vi "Get Channel Tag Path.vi"(11 "Waveform":waveform(dbl)) -> (3 "channel path":string)   [LabVIEW 2017, in "Logger.lvclass"]
uses:
  logger/Logger.lvclass
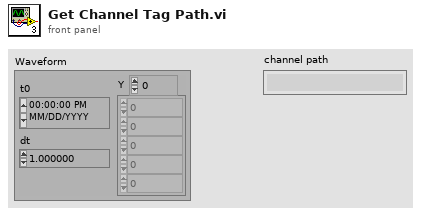
[diagram p1: front panel]
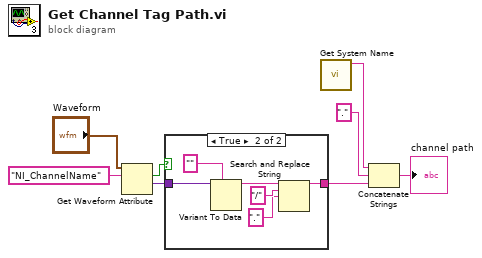
[diagram p0: block diagram]
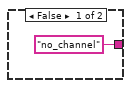
[diagram p2: hidden frame]
diagram:
  n1 = Get Waveform Attribute(6:"NI_ChannelName" ("name"), 7:"Waveform") -> (1:w7:variant, 2:w6:bool)  [unwired: 2 in, 2 out]
  n2 = case shown="True" w6 {
    tunnel: w7 -> [_ w15]
    tunnel: ["no_channel" ("result string") w12] -> w2
    frame False {
    }
    frame True {
      n3 = Variant To Data(type="" ("String"), Variant=w15) -> (data=w13:string)  [unwired: 1 in, 1 out]
      n4 = Search and Replace String(input string=w13, search string="/", replace string="." ("replace string (\"\")")) -> (result string=w12:string)  [unwired: 5 in, 3 out]
    }
  }
  n5 = call "Get System Name.vi"() -> ("name"=w1:string)  [unwired: 11 in]
  n6 = Concatenate Strings(w1, "." ("string"), w2) -> (→"channel path":string)
